vi "VS_XML - Main.vi"() -> ()   [LabVIEW 2014]
uses:
  xCE/_shared/tce_NewButton.ctl
  xCE/_shared/tce_OpenButton.ctl
  xCE/_shared/tce_SaveButton1.ctl
  xCE/_shared/tce_ExitButton.ctl
  xCE/_shared/StateVariables.ctl
  xCE/xceRootNode/xceRootNode.lvclass
  xCE/xceSubPanel/xceSubPanel.lvclass
  xCE/xceRootNode/RootInit.ctl
  xCE/xceSubPanel/SubPanel init.ctl
  <vilib>/NI/AMC/Message Queue.ctl
  <vilib>/NI/AMC/Message.ctl
  <vilib>/NI/Tools/Keyed Array/KeyedArray.ctl
  Veristand XML FPGA/FPGADMAChannelData/FPGADMAChannelData.lvclass
  xCE/_shared/menuSelection.ctl
  xCE/_shared/dropInfo.ctl
  xCE/xceRootNode/moveDirection.ctl
  xCE/xceDataNode/xceDataNode.lvclass
  xCE/_shared/replaceNode.ctl
  <vilib>/NI/AMC/Read Termination Message.vi
  <vilib>/NI/AMC/Create Single Message.vi
  <vilib>/NI/AMC/Update Message Routing Info.vi
  <vilib>/NI/AMC/Globals.vi
  <vilib>/NI/AMC/Send Message.vi
  <vilib>/NI/AMC/AMC.lvlib
  <vilib>/NI/Tools/Keyed Array/Tools_KeyedArray.lvlib
panel:
  in  "Tree":string(tree)="Node8"
  in  "New":T1
  in  "Exit":T2
  in  "Save":T3
  in  "Open":T4
  # "*Hold <Ctrl> and press <Up> or <Down> to move in the same \nhierarchy.\n*Hold <Ctrl> and use mouse to drag objects."
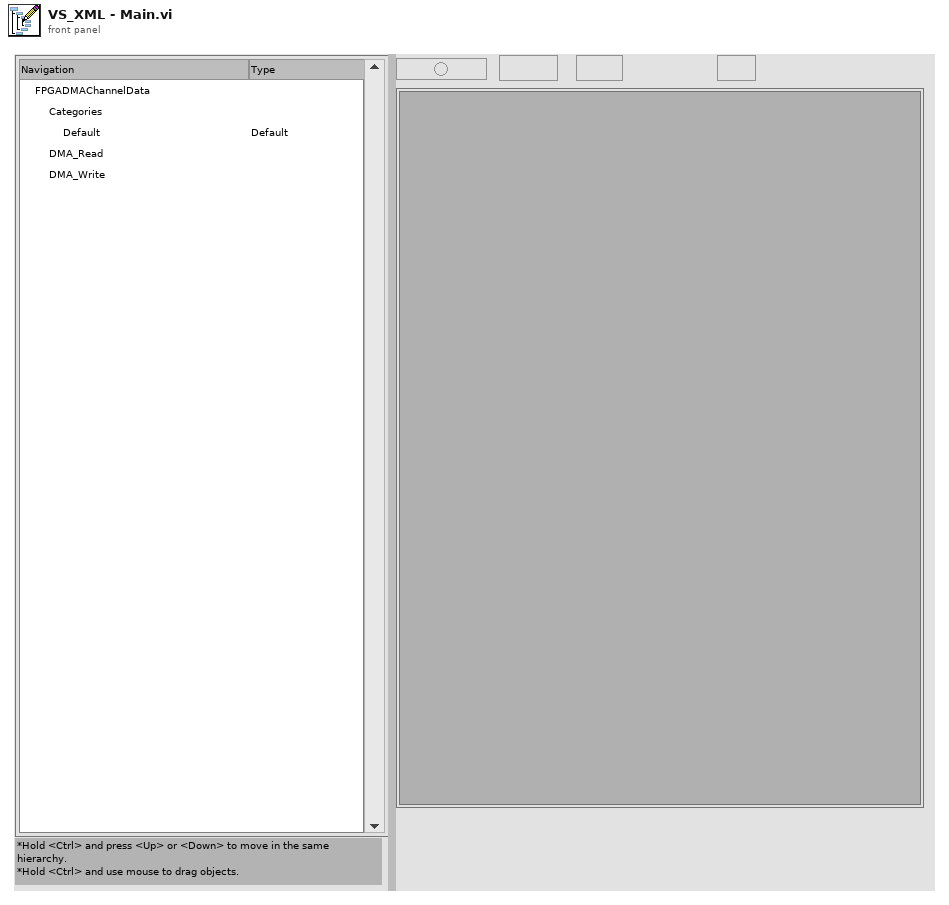
[diagram p1: front panel]
types:
  T1 = typedef "tce_NewButton.ctl" = bool
  T2 = typedef "tce_ExitButton.ctl" = bool
  T3 = typedef "tce_SaveButton1.ctl" = bool
  T4 = typedef "tce_OpenButton.ctl" = bool
  T5 = typedef "StateVariables.ctl" = cluster{"RootNode*":refnum<data-value>, "xceSubPanel":refnum<class "xceSubPanel.lvclass">}
  T6 = typedef "AMC.lvlib/Message Queue.ctl" = refnum<queue>
  T7 = typedef "menuSelection.ctl" = cluster{"menu Path":string, "Item Path":string}
  T8 = typedef "dropInfo.ctl" = cluster{"Item Path":string, "Drop Data":string}
  T9 = typedef "LVPoint32TypeDef.ctl" = cluster{"Horizontal":i32, "Vertical":i32}
  T10 = typedef "flatMenu.ctl" = cluster{"menuTag":string, "itemName":string}[]
  T11 = typedef "eventvkey.ctl" = enum16{"ASCII", "Enter", "Return", "Shift", "Ctrl", "Alt", "Cmd", "Opt", "Caps", "NumLock", "Clear", "Break", "Up", "Down", "Left", "Right", "Insert", "Delete", "Home", "End", "PageUp", "PageDown", "Escape", "Help", "Pause", "ScrollLock", "F1", "F2", "F3", "F4", "F5", "F6", "F7", "F8", "F9", "F10", "F11", "F12", "F13", "F14", "F15", "F16", "F17", "F18", "F19", "F20", "F21", "F22", "F23", "F24", "Play", "VolumeUp", "VolumeDown", "Mute", "Two Byte Char"}
  T12 = typedef "xceSubPanel.lvclass/SubPanel init.ctl" = cluster{"SubPanel*":refnum<vi>, "Front Panel*":refnum<vi>, "AMC*":T6}
  T13 = typedef "xceRootNode.lvclass/RootInit.ctl" = cluster{"TreeRef":refnum<vi>, "GlyphDirectory":path, "TopLevelMenu":refnum<k9>}
  T14 = typedef "xceRootNode.lvclass/moveDirection.ctl" = enum16{"Down", "Up"}
  T15 = typedef "replaceNode.ctl" = cluster{"ToReplaceNode*":refnum<data-value>, "Replace Class":string}
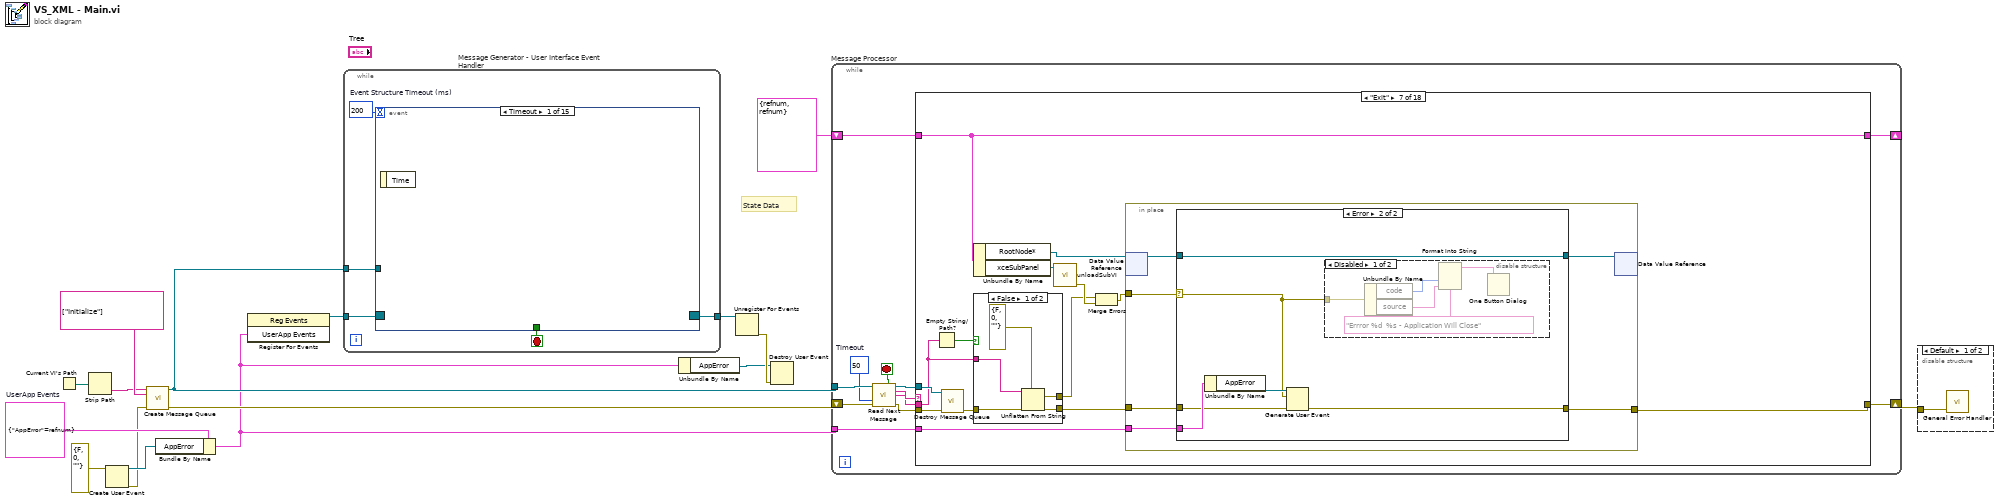
[diagram p0: block diagram]
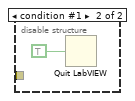
[diagram p2: hidden frame]
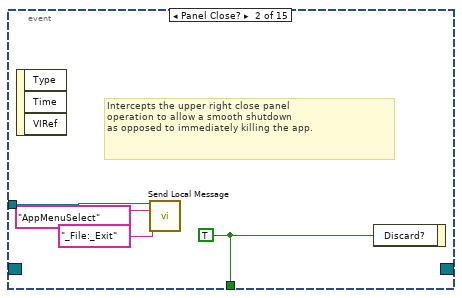
[diagram p3: hidden frame]
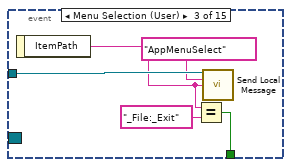
[diagram p4: hidden frame]
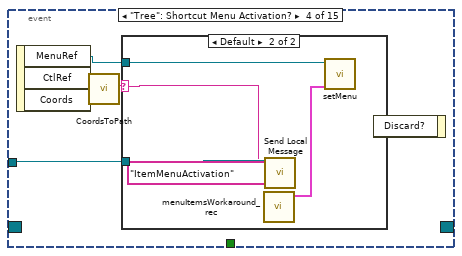
[diagram p5: hidden frame]
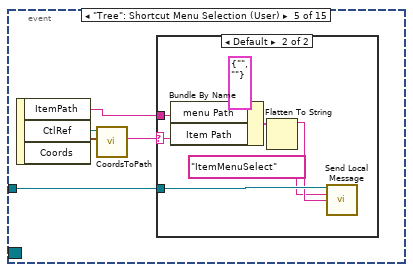
[diagram p7: hidden frame]
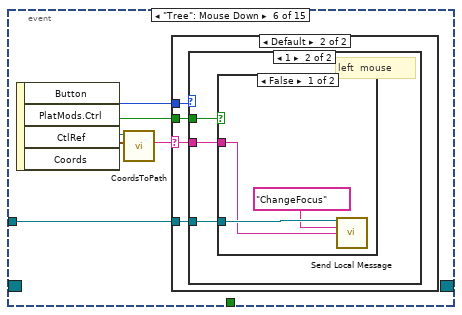
[diagram p9: hidden frame]
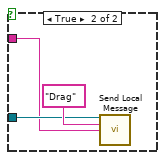
[diagram p12: hidden frame]
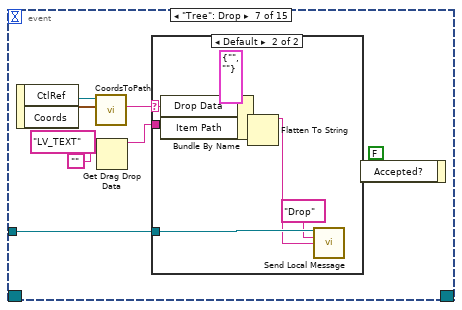
[diagram p13: hidden frame]
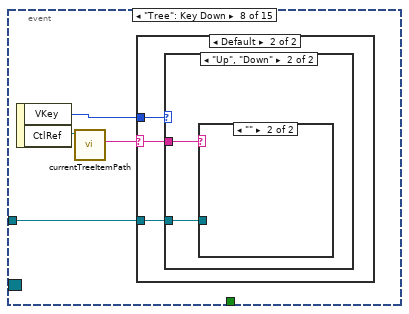
[diagram p15: hidden frame]
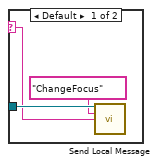
[diagram p18: hidden frame]
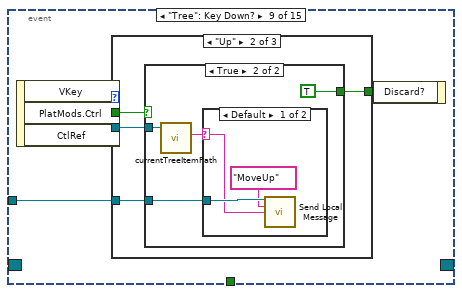
[diagram p19: hidden frame]
diagram:
  w8 = cluster{"AppError":refnum<user-event>} {"AppError"=refnum}  # UserApp Events
  # "State Data"
  n1 = Current VI's Path() -> (path=w12:path)
  n2 = Strip Path(path=w12) -> (name=w15:string)  [unwired: 1 out]
  n3 = Create User Event(user event datatype=errorcluster {"status"=FALSE, "code"=0, "source"=""} ("error constant")) -> (user event=w7:refnum<user-event>, error out=w6:errorcluster)  [unwired: 1 in]
  n4 = call <vilib>:"Create Message Queue.vi"("message queue name"=w15, "initial message names"=string[] ["Initialize"], "error in"=w6) -> ("message queue out"=w14:T6, "error out"=w13:errorcluster)  [unwired: 11 in]
  n5 = Bundle By Name(cluster=w8, "AppError"=w7) -> (w1:cluster{"AppError":refnum<user-event>})
  n6 = register-events(w1) -> (reference out=w5:refnum<event-registration>)  [unwired: 2 in, 1 out]
  n7 = while "Message Generator - User Interface Event Handler" {
    tunnel: w14 -> [w19]
    tunnel: w5 -> [w18]
    tunnel: [w17] -> w4
    stop <- w20 stop-if-true
    w21 = 200  # Event Structure Timeout (ms)
    n8 = event shown="[0] Timeout" {
      selector: w18 -> [_ _ _ _ _ _ _ _ _ _ _ _ _ _ _]
      dyn-events: [_ _ _ _ _ _ _ _ _ _ _ _ _ _ _] -> w17
      timeout: w21 -> [_ _ _ _ _ _ _ _ _ _ _ _ _ _ _]
      tunnel: [_ w25 w26 _ _ _ _ _ _ _ _ _ _ TRUE ("Discard?") TRUE ("Discard?")] -> w20
      tunnel: w19 -> [_ w23 w30 w33 w42 w54 w74 w88 w100 _ w131 w134 w137 w141 _]
      event Timeout {
        n9 = event-data() -> ()  [unwired: 2 out]
      }
      event Panel Close? {
        w25 = TRUE ("Discard?")
        # "Intercepts the upper right close panel\noperation to allow a smooth shutdown\nas opposed to immediately killing the app."
        n10 = event-data() -> ()  [unwired: 4 out]
        n11 = call <vilib>:"Send Local Message.vi"("message queue in"=w23, "message name"="AppMenuSelect", "message value"="_File:_Exit" ("Message Value")) -> ()  [unwired: 10 in, 3 out]
        n12 = event-data("Discard?"=w25) -> ()  [unwired: 1 in, 1 out]
      }
      event Menu Selection (User) {
        n13 = event-data() -> ("ItemPath"=w27:string)  [unwired: 1 out]
        n14 = Equal?(x=w27, y="_File:_Exit") -> (x = y?=w26:bool)
        n15 = call <vilib>:"Send Local Message.vi"("message queue in"=w30, "message name"="AppMenuSelect" ("Message Name"), "message value"=w27) -> ()  [unwired: 10 in, 3 out]
      }
      event "Tree": Shortcut Menu Activation? {
        n16 = event-data() -> ("MenuRef"=w32:refnum<k9>, "CtlRef"=w35:refnum<vi>, "Coords"=w34:T9)  [unwired: 1 out]
        n17 = call "CoordsToPath.vi"("Coords"=w34, "CtlRef"=w35) -> ("Item Path"=w31:string)  [unwired: 8 in, 1 out]
        n18 = case shown="Default" w31 {
          selector: w31 -> [_ w36]
          tunnel: w33 -> [_ w40]
          tunnel: w32 -> [_ w38]
          frame "" {
          }
          frame Default {
            n19 = call "menuItemsWorkaround_rec.vi"() -> ("flatMenu[]"=w37:T10)  [unwired: 10 in, 1 out]
            n20 = call <vilib>:"Send Local Message.vi"("message queue in"=w40, "message name"="ItemMenuActivation" ("Message Name"), "message value"=w36) -> ()  [unwired: 10 in, 3 out]
            n21 = call "setMenu.vi"("flatMenu[]"=w37, "MenuRef"=w38) -> ()  [unwired: 10 in]
          }
        }
        n22 = event-data() -> ()  [unwired: 2 in, 1 out]
      }
      event "Tree": Shortcut Menu Selection (User) {
        n23 = event-data() -> ("ItemPath"=w43:string, "CtlRef"=w44:refnum<vi>, "Coords"=w45:T9)  [unwired: 1 out]
        n24 = call "CoordsToPath.vi"("Coords"=w45, "CtlRef"=w44) -> ("Item Path"=w41:string)  [unwired: 8 in, 1 out]
        n25 = case shown="Default" w41 {
          selector: w41 -> [_ w46]
          tunnel: w43 -> [_ w51]
          tunnel: w42 -> [_ w49]
          frame "" {
          }
          frame Default {
            n26 = Bundle By Name(cluster=T7 {"menu Path"="", "Item Path"=""} ("menuSelection"), "menu Path"=w51, "Item Path"=w46) -> (w50:T7)
            n27 = Flatten To String(anything=w50) -> (data string=w48:string)  [unwired: 3 in, 2 out]
            n28 = call <vilib>:"Send Local Message.vi"("message queue in"=w49, "message name"="ItemMenuSelect" ("Message Name"), "message value"=w48) -> ()  [unwired: 10 in, 3 out]
          }
        }
      }
      event "Tree": Mouse Down {
        n29 = event-data() -> ("Button"=w56:u16, "PlatMods.Ctrl"=w55:bool, "CtlRef"=w58:refnum<vi>, "Coords"=w57:T9)  [unwired: 1 out]
        n30 = call "CoordsToPath.vi"("Coords"=w57, "CtlRef"=w58) -> ("Item Path"=w53:string)  [unwired: 8 in, 1 out]
        n31 = case shown="Default" w53 {
          selector: w53 -> [_ w59]
          tunnel: w56 -> [_ w62]
          tunnel: w55 -> [_ w61]
          tunnel: w54 -> [_ w60]
          frame "" {
          }
          frame Default {
            n32 = case shown="1" w62 {
              tunnel: w61 -> [_ w65]
              tunnel: w60 -> [_ w64]
              tunnel: w59 -> [_ w63]
              frame 2, Default {
                # "right mouse click"
              }
              frame 1 {
                # "left  mouse"
                n33 = case shown="False" w65 {
                  tunnel: w64 -> [w68 w70]
                  tunnel: w63 -> [w67 w69]
                  frame False {
                    n34 = call <vilib>:"Send Local Message.vi"("message queue in"=w68, "message name"="ChangeFocus" ("Message Name"), "message value"=w67) -> ()  [unwired: 10 in, 3 out]
                  }
                  frame True {
                    n35 = call <vilib>:"Send Local Message.vi"("message queue in"=w70, "message name"="Drag" ("Message Name"), "message value"=w69) -> ()  [unwired: 10 in, 3 out]
                  }
                }
              }
            }
          }
        }
      }
      event "Tree": Drop {
        n36 = event-data() -> ("CtlRef"=w77:refnum<vi>, "Coords"=w76:T9)  [unwired: 1 out]
        n37 = call "CoordsToPath.vi"("Coords"=w76, "CtlRef"=w77) -> ("Item Path"=w72:string)  [unwired: 8 in, 1 out]
        n38 = Get Drag Drop Data(8:"", 9:"LV_TEXT" ("data name")) -> (3:w75:string)  [unwired: 1 in, 1 out]
        n39 = case shown="Default" w72 {
          selector: w72 -> [_ w80]
          tunnel: w75 -> [_ w85]
          tunnel: w74 -> [_ w84]
          frame "" {
          }
          frame Default {
            n40 = Bundle By Name(cluster=T8 {"Item Path"="", "Drop Data"=""} ("Cluster"), "Drop Data"=w80, "Item Path"=w85) -> (w83:T8)
            n41 = Flatten To String(anything=w83) -> (data string=w82:string)  [unwired: 3 in, 2 out]
            n42 = call <vilib>:"Send Local Message.vi"("message queue in"=w84, "message name"="Drop" ("Message Name"), "message value"=w82) -> ()  [unwired: 10 in, 3 out]
          }
        }
        n43 = event-data("Accepted?"=FALSE) -> ()  [unwired: 1 in, 1 out]
      }
      event "Tree": Key Down {
        n44 = event-data() -> ("VKey"=w89:T11, "CtlRef"=w90:refnum<vi>)  [unwired: 1 out]
        n45 = call "currentTreeItemPath.vi"("TreeRef"=w90) -> ("treePath"=w87:string)  [unwired: 9 in, 1 out]
        n46 = case shown="Default" w87 {
          selector: w87 -> [_ w91]
          tunnel: w89 -> [_ w93]
          tunnel: w88 -> [_ w92]
          frame "" {
          }
          frame Default {
            n47 = case shown="\"Up\", \"Down\"" w93 {
              tunnel: w91 -> [_ w95]
              tunnel: w92 -> [_ w94]
              frame Default {
              }
              frame "Up", "Down" {
                n48 = case shown="\"\"" w95 {
                  selector: w95 -> [w96 _]
                  tunnel: w94 -> [w98 _]
                  frame Default {
                    n49 = call <vilib>:"Send Local Message.vi"("message queue in"=w98, "message name"="ChangeFocus" ("Message Name"), "message value"=w96) -> ()  [unwired: 10 in, 3 out]
                  }
                  frame "" {
                  }
                }
              }
            }
          }
        }
      }
      event "Tree": Key Down? {
        n50 = event-data() -> ("VKey"=w103:T11, "PlatMods.Ctrl"=w102:bool, "CtlRef"=w101:refnum<vi>)  [unwired: 1 out]
        n51 = case shown="\"Up\"" w103 {
          tunnel: w102 -> [_ w107 w118]
          tunnel: w101 -> [_ w106 w117]
          tunnel: w100 -> [_ w105 w116]
          tunnel: [_ w104 w115] -> w99
          frame Default {
          }
          frame "Up" {
            n52 = case shown="True" w107 {
              tunnel: w106 -> [_ w111]
              tunnel: w105 -> [_ w109]
              tunnel: [_ TRUE] -> w104
              frame False {
              }
              frame True {
                n53 = call "currentTreeItemPath.vi"("TreeRef"=w111) -> ("treePath"=w110:string)  [unwired: 9 in, 1 out]
                n54 = case shown="Default" w110 {
                  selector: w110 -> [w112 _]
                  tunnel: w109 -> [w114 _]
                  frame Default {
                    n55 = call <vilib>:"Send Local Message.vi"("message queue in"=w114, "message name"="MoveUp" ("Message Name"), "message value"=w112) -> ()  [unwired: 10 in, 3 out]
                  }
                  frame "" {
                  }
                }
              }
            }
          }
          frame "Down" {
            n56 = case shown="True" w118 {
              tunnel: w117 -> [_ w122]
              tunnel: w116 -> [_ w120]
              tunnel: [_ TRUE] -> w115
              frame False {
              }
              frame True {
                n57 = call "currentTreeItemPath.vi"("TreeRef"=w122) -> ("treePath"=w121:string)  [unwired: 9 in, 1 out]
                n58 = case shown="Default" w121 {
                  selector: w121 -> [w123 _]
                  tunnel: w120 -> [w125 _]
                  frame Default {
                    n59 = call <vilib>:"Send Local Message.vi"("message queue in"=w125, "message name"="MoveDown" ("Message Name"), "message value"=w123) -> ()  [unwired: 10 in, 3 out]
                  }
                  frame "" {
                  }
                }
              }
            }
          }
        }
        n60 = event-data("Discard?"=w99) -> ()  [unwired: 1 in, 1 out]
      }
      event "Tree": event type 3.0.x8000000b {
        n61 = event-data() -> ("VKey"=w127:T11)  [unwired: 1 out]
        n62 = case shown="\"Up\", \"Down\"" w127 {
          tunnel: [_ TRUE] -> w126
          frame Default {
          }
          frame "Up", "Down" {
          }
        }
        n63 = event-data("Discard?"=w126) -> ()  [unwired: 1 in, 1 out]
      }
      event Value Change {
        n64 = event-data() -> ()  [unwired: 2 out]
        n65 = call <vilib>:"Send Local Message.vi"("message queue in"=w131, "message name"="AppMenuSelect" ("Message Name"), "message value"="_File:_New" ("Message Value")) -> ()  [unwired: 10 in, 3 out]
      }
      event Value Change {
        n66 = event-data() -> ()  [unwired: 2 out]
        n67 = call <vilib>:"Send Local Message.vi"("message queue in"=w134, "message name"="AppMenuSelect" ("Message Name"), "message value"="_File:_Open" ("Message Value")) -> ()  [unwired: 10 in, 3 out]
      }
      event Value Change {
        n68 = event-data() -> ()  [unwired: 2 out]
        n69 = call <vilib>:"Send Local Message.vi"("message queue in"=w137, "message name"="AppMenuSelect" ("Message Name"), "message value"="_File:_Save" ("Message Value")) -> ()  [unwired: 10 in, 3 out]
      }
      event Value Change {
        n70 = event-data() -> ()  [unwired: 2 out]
        n71 = call <vilib>:"Send Local Message.vi"("message queue in"=w141, "message name"="AppMenuSelect" ("Message Name"), "message value"="_File:_Exit" ("Message Value")) -> ()  [unwired: 10 in, 3 out]
      }
      event User Event {
        # "Exit on any Error"
        n72 = event-data() -> ()  [unwired: 2 out]
      }
    }
  }
  n73 = Unbundle By Name(w1) -> ("AppError"=w2:refnum<user-event>)
  n74 = Unregister For Events(event registration refnum=w4) -> (error out=w3:errorcluster)  [unwired: 1 in]
  n75 = Destroy User Event(user event=w2, error in=w3) -> ()  [unwired: 1 out]
  n76 = while "Message Processor" {
    shift-left: w13 -> [w148]
    shift-right: [w152] -> w10
    tunnel: w14 -> [w149]
    shift-left: T5 {"RootNode*"=refnum, "xceSubPanel"=refnum} ("State Variables") -> [w154]
    shift-right: [w153] -> _
    tunnel: w1 -> [w143]
    stop <- w151 stop-if-true
    w146 = 50  # Timeout
    n77 = call <vilib>:"Read Next Message.vi"("message queue in"=w149, "timeout (1 ms)"=w146, "error in"=w148) -> ("exit process?"=w151:bool, "message queue out"=w150:T6, "message name"=w145:string, "message value"=w144:string, "error out"=w147:errorcluster)  [unwired: 5 in, 3 out]
    n78 = case shown="\"Exit\"" w145 {
      selector: w145 -> [_ _ w161 _ _ _ _ _ _ _ _ _ _ _ _ _ _ _]
      tunnel: [w156 w158 w163 w167 w173 w192 w218 w251 w254 w296 w308 w352 w362 w374 w385 w396 w416 w449] -> w153
      tunnel: w154 -> [w156 w158 w163 w167 w173 w193 w218 w251 w254 w296 w308 w353 w362 w374 w385 w396 w416 w451]
      tunnel: w150 -> [_ _ _ w169 _ w185 w219 _ w255 _ w303 _ _ _ _ _ _ w439]
      tunnel: w147 -> [w155 w157 w162 w164 w172 w194 w220 w250 w259 w293 w315 w350 w360 w378 w387 w398 w420 w452]
      tunnel: [w155 w157 w162 errorcluster {"status"=FALSE, "code"=0, "source"=""} ("error out") w172 w178 w210 w250 w256 w292 w305 w351 w359 w369 w386 w397 w417 w440] -> w152
      tunnel: w144 -> [_ _ _ _ _ _ w212 _ w260 w294 w313 w355 w361 w376 w388 w399 w419 w453]
      tunnel: w143 -> [_ _ _ _ _ _ w211 _ _ _ _ _ _ _ _ _ _ _]
      frame "---------- Framework Operations ----------" {
        # "Dummy case to add a seperator in the Case Structure menu"
      }
      frame "", "Idle" {
      }
      frame "Missing Message Handler", Default {
        # "Call this case if a message is received that is not handled \nby any other case. Typically this is a programming error\nas a result of a typo or unhandled message/missing message handler."
        n79 = Format Into String(format string="DevError: Missing message handler for '%s\" message." ("message"), w161) -> (resulting string=w159:string)  [unwired: 2 in, 1 out]
        n80 = One Button Dialog(message=w159) -> ()  [unwired: 2 out]
      }
      frame "Error" {
        # "Proceed to Exit - Remove this if it is\nnot appropriate for the General Error case"
        n81 = disable-structure shown="Enabled" {
          disable-tunnel: w164 -> [w171 _]
          frame Disabled {
            n82 = call <vilib>:"Simple Error Handler.vi"("error in (no error)"=w171) -> ()  [unwired: 1 in, 8 out]
          }
          frame Enabled {
          }
        }
        n83 = Unbundle By Name(w167) -> ("xceSubPanel"=w166:refnum<class "xceSubPanel.lvclass">)
        n84 = call "unloadSubVI.vi"("SubPanel in"=w166) -> ()  [unwired: 8 in, 3 out]
        n85 = Flatten To String(anything=w164) -> (data string=w165:string)  [unwired: 3 in, 2 out]
        n86 = call <vilib>:"Send Local Message.vi"("message queue in"=w169, "message name"="Exit", "message value"=w165) -> ()  [unwired: 10 in, 3 out]
      }
      frame "---------- Generic Operations ----------" {
        # "Dummy case to add a seperator in the Case Structure menu"
      }
      frame "Initialize" {
        n87 = Current VI's Path() -> (path=w175:path)
        n88 = disable-structure shown="RUN_TIME_ENGINE==True" {
          disable-tunnel: w175 -> [w199 w202]
          disable-tunnel: [w200 w205] -> w174
          frame condition #0 (active) {
            n89 = Strip Path(path=w199) -> (stripped path=w198:path)  [unwired: 1 out]
            n90 = Build Path(base path=w198, name or relative path="Veristand XML FPGA\\_Shared\\Glyphs") -> (appended path=w200:path)
          }
          frame condition #1 {
            n91 = Strip Path(path=w202) -> (stripped path=w203:path)  [unwired: 1 out]
            n92 = Strip Path(path=w203) -> (stripped path=w204:path)  [unwired: 1 out]
            n93 = Build Path(base path=w204, name or relative path="data") -> (appended path=w205:path)
          }
        }
        n94 = control-ref of="This VI"() -> (w188:refnum<vi>)
        n95 = control-ref of="Tree"() -> (w196:refnum<vi>)
        n96 = control-ref of="Sub Panel"() -> (w189:refnum<vi>)
        n97 = property class="VI"(reference=w188) -> ("Panel"=w187:refnum<vi>)  [unwired: 1 in, 2 out]
        n98 = Current VI's Menubar() -> (w183:refnum<k9>)
        n99 = Bundle By Name(cluster=T13 {"TreeRef"=refnum, "GlyphDirectory"=path "", "TopLevelMenu"=refnum} ("InitRoot"), "TreeRef"=w196, "TopLevelMenu"=w183, "GlyphDirectory"=w174) -> (w195:T13)
        n100 = Bundle By Name(cluster=T12 {"SubPanel*"=refnum, "Front Panel*"=refnum, "AMC*"=refnum} ("SubPanel init"), "AMC*"=w185, "SubPanel*"=w189, "Front Panel*"=w187) -> (w186:T12)
        n101 = call-dynamic "InitializeRoot.vi"("error in (no error)"=w194, "InitRoot"=w195, "xceRootNode in"=refnum<class "FPGADMAChannelData.lvclass"> refnum ("FPGADMAChannelData.lvclass")) -> ("error out"=w184:errorcluster, "RootNode*"=w179:refnum<data-value>)  [unwired: 7 in]
        n102 = call "Initialize.vi"("error in"=w184, "SubPanel init"=w186, "SubPanel in"=refnum<class "xceSubPanel.lvclass"> refnum ("xceSubPanel.lvclass")) -> ("error out"=w180:errorcluster, "SubPanel out"=w182:refnum<class "xceSubPanel.lvclass">)  [unwired: 7 in]
        n103 = call "loadSubVI.vi"("error in"=w180, "Node Path"="Node0", "RootNode*"=w179, "SubPanel in"=w182) -> ("error out"=w178:errorcluster, "SubPanel"=w181:refnum<class "xceSubPanel.lvclass">)  [unwired: 6 in]
        n104 = Bundle By Name(cluster=w193, "xceSubPanel"=w181, "RootNode*"=w179) -> (w192:T5)
      }
      frame "Exit" {
        n105 = Empty String/Path?(string/path=w212) -> (empty?=w213:bool)
        n106 = call <vilib>:"Destroy Message Queue.vi"("message queue in"=w219, "error in"=w220) -> ("error out"=w215:errorcluster)  [unwired: 11 in, 2 out]
        n107 = case shown="False" w213 {
          tunnel: w215 -> [w225 w227]
          tunnel: w212 -> [w224 _]
          tunnel: [w222 errorcluster {"status"=FALSE, "code"=0, "source"=""} ("error out")] -> w207
          tunnel: [w221 w227] -> w214
          frame False {
            n108 = Unflatten From String(type=errorcluster {"status"=FALSE, "code"=0, "source"=""} ("error out"), binary string=w224, error in (no error)=w225) -> (value=w222:errorcluster, error out=w221:errorcluster)  [unwired: 2 in, 1 out]
          }
          frame True {
          }
        }
        n109 = Unbundle By Name(w218) -> ("RootNode*"=w216:refnum<data-value>, "xceSubPanel"=w217:refnum<class "xceSubPanel.lvclass">)
        n110 = call "unloadSubVI.vi"("SubPanel in"=w217) -> ("error out"=w208:errorcluster)  [unwired: 8 in, 2 out]
        n111 = Merge Errors(w207, w208) -> (w209:errorcluster)
        n112 = in-place {
          in-place-border: w214 -> [w231]
          in-place-border: [w230] -> w210
          in-place-border: w209 -> [w229]
          in-place-border: w211 -> [w228]
          n113 = in-place-dvr #1(w216) -> (w233:refnum<class "xceRootNode.lvclass">)  [unwired: 1 out]
          n114 = case shown="Error" w229 {
            selector: w229 -> [_ w238]
            tunnel: w233 -> [w237 w243]
            tunnel: [w236 w243] -> w232
            tunnel: w231 -> [w235 w240]
            tunnel: [w234 w239] -> w230
            tunnel: w228 -> [_ w242]
            frame No Error {
              n115 = call "promptSaveNodes.vi"("error in (no error)"=w235, "xceRootNode in"=w237) -> ("error out"=w234:errorcluster, "xceRootNode out"=w236:refnum<class "xceRootNode.lvclass">)  [unwired: 7 in, 1 out]
            }
            frame Error {
              n116 = Unbundle By Name(w242) -> ("AppError"=w241:refnum<user-event>)
              n117 = Generate User Event(user event=w241, event data cluster=w238, error in=w240) -> (error out=w239:errorcluster)  [unwired: 1 in, 1 out]
              n118 = disable-structure shown="Disabled" {
                disable-tunnel: w238 -> [w245 w249]
                frame Disabled {
                  n119 = Unbundle By Name(w245) -> ("code"=w247:i32, "source"=w244:string)
                  n120 = Format Into String(format string="Errror %d  %s - Application Will Close" ("initial string"), w247, w244) -> (resulting string=w248:string)  [unwired: 2 in, 1 out]
                  n121 = One Button Dialog(message=w248) -> ()  [unwired: 1 in, 1 out]
                }
                frame Enabled {
                  n122 = call <vilib>:"Simple Error Handler.vi"("error in (no error)"=w249) -> ()  [unwired: 4 in, 5 out]
                }
              }
            }
          }
          n123 = in-place-dvr #1(w232) -> ()  [unwired: 2 out]
        }
      }
      frame "---------- Application Operations ----------" {
        # "Dummy case to add a seperator in the Case Structure menu"
      }
      frame "AppMenuSelect" {
        n124 = Unbundle By Name(w254) -> ("xceSubPanel"=w253:refnum<class "xceSubPanel.lvclass">, "RootNode*"=w261:refnum<data-value>)
        n125 = in-place {
          in-place-border: w260 -> [w288]
          in-place-border: w259 -> [w287]
          in-place-border: [w286] -> w257
          in-place-border: [w285] -> w258
          n126 = in-place-dvr #2(w261) -> (w290:refnum<class "xceRootNode.lvclass">)  [unwired: 1 out]
          n127 = call-dynamic "AppMenuSelection.vi"("error in (no error)"=w287, "Menu Selection in"=w288, "xceRootNode in"=w290) -> ("error out"=w286:errorcluster, "New Message"=w285:string, "xceRootNode out"=w289:refnum<class "xceRootNode.lvclass">)  [unwired: 5 in, 1 out]
          n128 = in-place-dvr #2(w289) -> (w252:refnum<data-value>)  [unwired: 1 out]
        }
        n129 = case shown="\"refresh\"" w258 {
          selector: w258 -> [w265 w269 _ _]
          tunnel: w257 -> [w264 w267 w274 w284]
          tunnel: [w263 w270 w272 w284] -> w256
          tunnel: w255 -> [w262 w271 _ _]
          tunnel: w253 -> [_ w268 _ _]
          tunnel: w252 -> [_ _ _ _]
          frame Default {
            n130 = call <vilib>:"Send Local Message.vi"("message queue in"=w262, "message name"=w265, "error in"=w264) -> ("error out"=w263:errorcluster)  [unwired: 10 in, 2 out]
          }
          frame "Initialize" {
            n131 = call "unloadSubVI.vi"("error in"=w267, "SubPanel in"=w268) -> ("error out"=w266:errorcluster)  [unwired: 7 in, 2 out]
            n132 = call <vilib>:"Send Local Message.vi"("message queue in"=w271, "message name"=w269, "error in"=w266) -> ("error out"=w270:errorcluster)  [unwired: 10 in, 2 out]
          }
          frame "refresh" {
            # "Ignore error \n537053"
            # "Force Refresh on Panel Controls of the Panel VI"
            n133 = call <vilib>:"Send Local Message.vi"("receiver process (\"\" - local)"="FPGADMAChannelDataUI.vi" ("Process (\"\" - local)"), "message name"="Initialize" ("Message Name"), "error in"=w274) -> ("error out"=w273:errorcluster)  [unwired: 10 in, 2 out]
            n134 = case shown="Error" w273 {
              selector: w273 -> [w277 w280]
              tunnel: [w277 w278] -> w272
              frame No Error {
              }
              frame Error {
                n135 = Unbundle By Name(w280) -> ("code"=w283:i32)
                n136 = Equal?(x=w283, y=537053) -> (x = y?=w281:bool)
                n137 = Select(t=errorcluster {"status"=FALSE, "code"=0, "source"=""}, s=w281, f=w280) -> (s? t:f=w278:errorcluster)
              }
            }
          }
          frame "" {
          }
        }
      }
      frame "ItemMenuActivation" {
        n138 = Unbundle By Name(w296) -> ("RootNode*"=w295:refnum<data-value>)
        n139 = in-place {
          in-place-border: w294 -> [w298]
          in-place-border: w293 -> [w300]
          in-place-border: [w299] -> w292
          in-place-border: [w297] -> w291
          n140 = in-place-dvr #3(w295) -> (w302:refnum<class "xceRootNode.lvclass">)  [unwired: 1 out]
          n141 = call "NodeMenuActivation.vi"("error in (no error)"=w300, "Node Path"=w298, "xceRootNode in"=w302) -> ("error out"=w299:errorcluster, "flatMenu[]"=w297:T10, "xceRootNode out"=w301:refnum<class "xceRootNode.lvclass">)  [unwired: 6 in]
          n142 = in-place-dvr #3(w301) -> ()  [unwired: 2 out]
        }
        n143 = call "menuItemsWorkaround_send.vi"("flatMenu[]"=w291) -> ()  [unwired: 11 in]
      }
      frame "ItemMenuSelect" {
        n144 = Unflatten From String(type=T7 {"menu Path"="", "Item Path"=""} ("menuSelection"), binary string=w313, error in (no error)=w315) -> (value=w312:T7, error out=w309:errorcluster)  [unwired: 2 in, 1 out]
        n145 = Unbundle By Name(w308) -> ("RootNode*"=w310:refnum<data-value>)
        n146 = Unbundle By Name(w312) -> ("menu Path"=w311:string, "Item Path"=w304:string)
        n147 = in-place {
          in-place-border: w311 -> [w348]
          in-place-border: w304 -> [w347]
          in-place-border: w309 -> [w345]
          in-place-border: [w344] -> w306
          in-place-border: [w342] -> _
          n148 = in-place-dvr #4(w310) -> (w346:refnum<class "xceRootNode.lvclass">)  [unwired: 1 out]
          n149 = call "NodeMenuSelection.vi"("error in (no error)"=w345, "Item Path in"=w347, "Menu Path in"=w348, "xceRootNode in"=w346) -> ("error out"=w344:errorcluster, "Menu Path out"=w342:string, "xceRootNode out"=w343:refnum<class "xceRootNode.lvclass">)  [unwired: 4 in, 1 out]
          n150 = in-place-dvr #4(w343) -> (w307:refnum<data-value>)  [unwired: 1 out]
        }
        n151 = disable-structure shown="Enabled" {
          disable-tunnel: w307 -> [w326 _]
          disable-tunnel: w306 -> [w325 w341]
          disable-tunnel: [w319 w341] -> w305
          disable-tunnel: w304 -> [w321 _]
          disable-tunnel: w303 -> [w320 _]
          frame Enabled {
            # "Rename Packet to avoid name assignign"
            n152 = To More Specific Class(target class=refnum<data-value> refnum ("data value reference"), reference=w326, error in=w325) -> (specific class reference=w323:refnum<data-value>, error out=w322:errorcluster)
            n153 = in-place {
              in-place-border: w322 -> [w337]
              in-place-border: [w340] -> w317
              in-place-border: w321 -> [w336]
              in-place-border: [w335] -> w318
              in-place-border: [w334] -> w316
              n154 = in-place-dvr #5(w323) -> (w338:refnum<class "FPGADMAChannelData.lvclass">)  [unwired: 1 out]
              n155 = call "Check Node Class Name.vi"("error in (no error)"=w337, "Node Path"=w336, "FPGADMAChannelData in"=w338) -> ("error out"=w340:errorcluster, "Found Class?"=w334:bool, "Node*"=w335:refnum<data-value>, "FPGADMAChannelData out"=w339:refnum<class "FPGADMAChannelData.lvclass">)  [unwired: 5 in]
              n156 = in-place-dvr #5(w339) -> ()  [unwired: 2 out]
            }
            n157 = case shown="True" w316 {
              tunnel: w320 -> [_ w331]
              tunnel: [w327 w330] -> w319
              tunnel: w318 -> [_ w329]
              tunnel: w317 -> [w327 w328]
              frame False {
              }
              frame True {
                n158 = Flatten To String(anything=w329) -> (data string=w332:string)  [unwired: 3 in, 2 out]
                n159 = call <vilib>:"Send Local Message.vi"("message queue in"=w331, "message name"="refreshNode" ("Message Name"), "message value"=w332, "error in"=w328) -> ("error out"=w330:errorcluster)  [unwired: 9 in, 2 out]
              }
            }
          }
          frame Disabled {
          }
        }
      }
      frame "ChangeFocus" {
        n160 = Unbundle By Name(w353) -> ("RootNode*"=w356:refnum<data-value>, "xceSubPanel"=w358:refnum<class "xceSubPanel.lvclass">)
        n161 = call "unloadSubVI.vi"("error in"=w350, "SubPanel in"=w358) -> ("error out"=w349:errorcluster, "SubPanel out"=w357:refnum<class "xceSubPanel.lvclass">)  [unwired: 7 in, 1 out]
        n162 = call "loadSubVI.vi"("error in"=w349, "Node Path"=w355, "RootNode*"=w356, "SubPanel in"=w357) -> ("error out"=w351:errorcluster, "SubPanel"=w354:refnum<class "xceSubPanel.lvclass">)  [unwired: 6 in]
        n163 = Bundle By Name(cluster=w353, "xceSubPanel"=w354) -> (w352:T5)
      }
      frame "Drag" {
        n164 = Unbundle By Name(w362) -> ("RootNode*"=w363:refnum<data-value>)
        n165 = in-place {
          in-place-border: w361 -> [w366]
          in-place-border: w360 -> [w365]
          in-place-border: [w364] -> w359
          n166 = in-place-dvr #6(w363) -> (w368:refnum<class "xceRootNode.lvclass">)  [unwired: 1 out]
          n167 = call "dragNode.vi"("error in (no error)"=w365, "Node Path"=w366, "xceRootNode in"=w368) -> ("error out"=w364:errorcluster, "xceRootNode out"=w367:refnum<class "xceRootNode.lvclass">)  [unwired: 7 in]
          n168 = in-place-dvr #6(w367) -> ()  [unwired: 2 out]
        }
      }
      frame "Drop" {
        n169 = Unflatten From String(type=T8 {"Item Path"="", "Drop Data"=""} ("Cluster"), binary string=w376, error in (no error)=w378) -> (value=w373:T8, error out=w370:errorcluster)  [unwired: 2 in, 1 out]
        n170 = Unbundle By Name(w374) -> ("RootNode*"=w375:refnum<data-value>)
        n171 = Unbundle By Name(w373) -> ("Item Path"=w372:string, "Drop Data"=w371:string)
        n172 = in-place {
          in-place-border: w372 -> [w382]
          in-place-border: w371 -> [w381]
          in-place-border: w370 -> [w380]
          in-place-border: [w379] -> w369
          n173 = in-place-dvr #7(w375) -> (w384:refnum<class "xceRootNode.lvclass">)  [unwired: 1 out]
          n174 = call "dropNode.vi"("error in (no error)"=w380, "Drop Node Path"=w381, "Drag Node Path"=w382, "xceRootNode in"=w384) -> ("error out"=w379:errorcluster, "xceRootNode out"=w383:refnum<class "xceRootNode.lvclass">)  [unwired: 6 in]
          n175 = in-place-dvr #7(w383) -> ()  [unwired: 2 out]
        }
      }
      frame "MoveDown" {
        n176 = Unbundle By Name(w385) -> ("RootNode*"=w389:refnum<data-value>)
        n177 = in-place {
          in-place-border: w388 -> [w394]
          in-place-border: w387 -> [w392]
          in-place-border: [w391] -> w386
          n178 = in-place-dvr #8(w389) -> (w395:refnum<class "xceRootNode.lvclass">)  [unwired: 1 out]
          n179 = call "moveNode.vi"("error in (no error)"=w392, "Direction"=moveDirection."Down", "Node Path"=w394, "xceRootNode in"=w395) -> ("error out"=w391:errorcluster, "xceRootNode out"=w390:refnum<class "xceRootNode.lvclass">)  [unwired: 6 in]
          n180 = in-place-dvr #8(w390) -> ()  [unwired: 2 out]
        }
      }
      frame "MoveUp" {
        n181 = Unbundle By Name(w396) -> ("RootNode*"=w400:refnum<data-value>)
        n182 = in-place {
          in-place-border: w399 -> [w405]
          in-place-border: w398 -> [w403]
          in-place-border: [w402] -> w397
          n183 = in-place-dvr #9(w400) -> (w406:refnum<class "xceRootNode.lvclass">)  [unwired: 1 out]
          n184 = call "moveNode.vi"("error in (no error)"=w403, "Direction"=moveDirection."Up", "Node Path"=w405, "xceRootNode in"=w406) -> ("error out"=w402:errorcluster, "xceRootNode out"=w401:refnum<class "xceRootNode.lvclass">)  [unwired: 6 in]
          n185 = in-place-dvr #9(w401) -> ()  [unwired: 2 out]
        }
      }
      frame "refreshNode" {
        n186 = Unflatten From String(type=refnum<data-value> refnum ("DataNode*"), binary string=w419, error in (no error)=w420) -> (value=w415:refnum<data-value>, error out=w414:errorcluster)  [unwired: 2 in, 1 out]
        n187 = Unbundle By Name(w416) -> ("RootNode*"=w421:refnum<data-value>)
        n188 = in-place {
          in-place-border: w414 -> [w428]
          in-place-border: [w429] -> w413
          in-place-border: [w428] -> w412
          n189 = in-place-dvr #10(w415) -> (w429:refnum<class "xceDataNode.lvclass">)  [unwired: 1 out]
          n190 = in-place-dvr #10(w429) -> (w411:refnum<data-value>)  [unwired: 1 out]
        }
        n191 = call "Check Downcast (Multiple).vi"("error in (no error)"=w412, "xceDataNode In"=w413) -> ("error out"=w410:errorcluster, "Ok?"=w408:bool)  [unwired: 7 in, 1 out]
        n192 = case shown="True" w408 {
          tunnel: w411 -> [w423 w426]
          tunnel: w410 -> [w422 w427]
          tunnel: [w422 w424] -> w409
          tunnel: [w423 w425] -> w407
          frame False {
          }
          frame True {
            n193 = call "Rename Child Nodes to Default Class Name.vi"("error in (no error)"=w427, "DataNode*"=w426) -> ("error out"=w424:errorcluster, "DataNode* Out"=w425:refnum<data-value>)  [unwired: 8 in]
          }
        }
        n194 = in-place {
          in-place-border: [w432] -> w417
          in-place-border: w407 -> [w431]
          in-place-border: w409 -> [w430]
          n195 = in-place-dvr #11(w421) -> (w434:refnum<class "xceRootNode.lvclass">)  [unwired: 1 out]
          n196 = call-dynamic "refreshNode.vi"("error in (no error)"=w430, "DataNode*"=w431, "xceRootNode in"=w434) -> ("error out"=w432:errorcluster, "xceRootNode out"=w433:refnum<class "xceRootNode.lvclass">)  [unwired: 7 in]
          n197 = in-place-dvr #11(w433) -> ()  [unwired: 2 out]
        }
      }
      frame "replaceNode" {
        n198 = Unflatten From String(type=T15 {"ToReplaceNode*"=refnum, "Replace Class"=""} ("replaceNode"), binary string=w453, error in (no error)=w452) -> (value=w444:T15, error out=w445:errorcluster)  [unwired: 2 in, 1 out]
        n199 = Unbundle By Name(w444) -> ("ToReplaceNode*"=w443:refnum<data-value>, "Replace Class"=w442:string)
        n200 = Unbundle By Name(w451) -> ("RootNode*"=w441:refnum<data-value>, "xceSubPanel"=w455:refnum<class "xceSubPanel.lvclass">)
        n201 = call "replaceNodes.vi"("error in (no error)"=w445, "Replace Class"=w442, "ToReplaceNode*"=w443, "RootNode* in"=w441) -> ("error out"=w446:errorcluster, "ReplaceNode*"=w436:refnum<data-value>)  [unwired: 5 in, 1 out]
        n202 = call "unloadSubVI.vi"("error in"=w446, "SubPanel in"=w455) -> ("error out"=w448:errorcluster, "SubPanel out"=w454:refnum<class "xceSubPanel.lvclass">)  [unwired: 7 in, 1 out]
        n203 = Flatten To String(anything=w436) -> (data string=w435:string)  [unwired: 3 in, 2 out]
        n204 = call "loadSubVIfromRef.vi"("error in (no error)"=w448, "DataNode*"=w436, "RootNode*"=w441, "xceSubPanel in"=w454) -> ("error out"=w437:errorcluster, "xceSubPanel out"=w450:refnum<class "xceSubPanel.lvclass">)  [unwired: 6 in]
        n205 = Bundle By Name(cluster=w451, "xceSubPanel"=w450) -> (w449:T5)
        n206 = call <vilib>:"Send Local Message.vi"("message queue in"=w439, "message name"="refreshNode" ("Message Name"), "message value"=w435, "error in"=w437) -> ("error out"=w440:errorcluster)  [unwired: 9 in, 2 out]
      }
    }
  }
  n207 = disable-structure shown="Default" {
    disable-tunnel: w10 -> [w456 _]
    frame condition #0 (active) {
      n208 = call <vilib>:"General Error Handler.vi"("error in (no error)"=w456) -> ()  [unwired: 10 in, 5 out]
    }
    frame condition #1 {
      n209 = Quit LabVIEW(quit? (T)=TRUE) -> ()
    }
  }
